vi "Interpolate R to T.vi"(7 "CHANNEL":i32, 8 "RESISTANCE (OHMS)":dbl, 9 "FILE INFO":T1(array[cluster]), 10 "R/T POINTS":cluster{dbl, dbl}[][](array[cluster]), 11 "CONFIGURATION CLUSTER":T2) -> (1 "TEMPERATURE":dbl, 2 "TEMPERATURE UNIT":string, 3 "UNMODIFIED CONFIGURATION CLUSTER":T2, 5 "R PAST CALIBRATION RANGE":bool)   [LabVIEW 2012]
doc: "Calculates temperature from the given\nor measured resistance. Uses the \nchannel's calibration curve for inter-\npolation."
panel:
  # "Interpolate R to T.vi"
  # "This is the \"direct temperature display VI\".  It requires the file info array of clusters and the R/T points 2-dimensional array of clusters. Both clusters are obtained by running \"read all RT calibration files.vi\". \n\nIndependent of the sign of the temperature coefficient of the sensor, the R values must be in ascending order. If the input value R is lower than R of the first breakpoint, or if it higher than the R of the last breakpoint, the first or last breakpoint temperature is returned and the \"R past calibration range\" indicator is set true.\n\nInstead of resistances, the calibration file can list breakpoints using log(R). This alternative must have been specified in the information file."
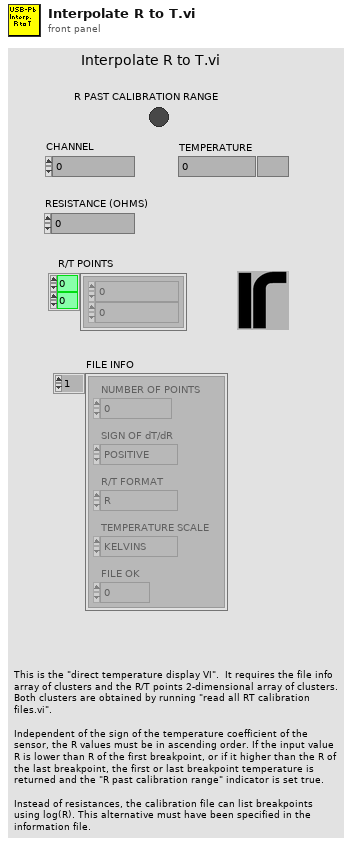
[diagram p1: front panel]
types:
  T1 = cluster{"NUMBER OF POINTS":i32, "SIGN OF dT/dR":enum16{"POSITIVE", "NEGATIVE"}, "R/T FORMAT ":enum16{"R", "LOG(R)"}, "TEMPERATURE SCALE":enum16{"KELVINS", "CELSIUS"}, "FILE OK":i32}[]
  T2 = cluster{"VISA RESOURCE":refnum<visa-resource-name>, "PICOBUS ADDRESS":u8, "DISABLE AL":u8, "REMOTE":u8, "INPUT":u8, "CHANNEL":u8, "RANGE":u8, "EXCITATION":u8, "DISPLAY":u8, "DIGITAL REFERENCE":u16, "SET POINT":dbl, "PROP GAIN":u8, "INTG":u8, "DERIV":u8, "POWER BIAS":u8, "POWER RANGE":u8, "INFO STRING":string, "HEATER RESISTANCE":dbl, "INTERVAL":u8, " SENSOR dR/dT":u8}
  T3 = cluster{"NUMBER OF POINTS":i32, "SIGN OF dT/dR":enum16{"POSITIVE", "NEGATIVE"}, "R/T FORMAT ":enum16{"R", "LOG(R)"}, "TEMPERATURE SCALE":enum16{"KELVINS", "CELSIUS"}, "FILE OK":i32}
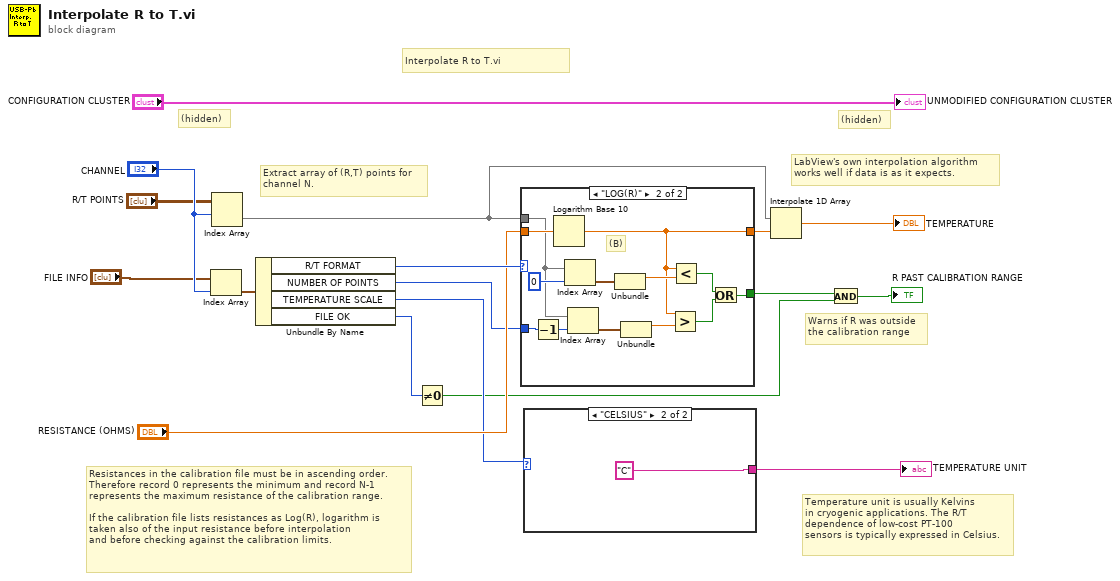
[diagram p0: block diagram]
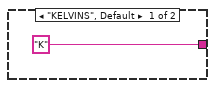
[diagram p2: hidden frame]
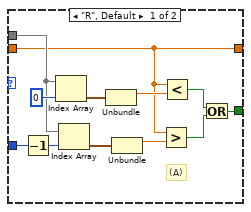
[diagram p3: hidden frame]
diagram:
  # "Resistances in the calibration file must be in ascending order.\nTherefore record 0 represents the minimum and record N-1\nrepresents the maximum resistance of the calibration range.\n\nIf the calibration file lists resistances as Log(R), logarithm is\ntaken also of the input resistance before interpolation\nand before checking against the calibration limits."
  # "LabView's own interpolation algorithm\nworks well if data is as it expects."
  # "Temperature unit is usually Kelvins\nin cryogenic applications. The R/T\ndependence of low-cost PT-100\nsensors is typically expressed in Celsius."
  # "Warns if R was outside\nthe calibration range"
  # "Extract array of (R,T) points for \nchannel N."
  # "(hidden)"
  # "(hidden)"
  # "Interpolate R to T.vi"
  n1 = Index Array(array="FILE INFO", index="CHANNEL") -> (element=w15:T3)
  n2 = Index Array(array="R/T POINTS", index (row)="CHANNEL") -> (element=w10:cluster{dbl, dbl}[])  [unwired: 1 in]
  n3 = Unbundle By Name(w15) -> ("R/T FORMAT"=w13:enum16{"R", "LOG(R)"}, "NUMBER OF POINTS"=w11:i32, "TEMPERATURE SCALE"=w8:enum16{"KELVINS", "CELSIUS"}, "FILE OK"=w5:i32)
  n4 = Not Equal To 0?(x=w5) -> (x != 0?=w1:bool)
  n5 = case shown="\"LOG(R)\"" w13 {
    tunnel: "RESISTANCE (OHMS)" -> [w19 w42]
    tunnel: [w19 w31] -> w14
    tunnel: w11 -> [w21 w33]
    tunnel: w10 -> [w20 w32]
    tunnel: [w18 w30] -> w3
    frame "R", Default {
      # "(A)"
      n6 = Decrement(x=w21) -> (x-1=w26:i32)
      n7 = Index Array(array=w20, index=0) -> (element=w27:cluster{dbl, dbl})
      n8 = Index Array(array=w20, index=w26) -> (element=w28:cluster{dbl, dbl})
      n9 = Unbundle(w27) -> (w23:dbl)  [unwired: 1 out]
      n10 = Unbundle(w28) -> (w22:dbl)  [unwired: 1 out]
      n11 = Greater?(x=w19, y=w22) -> (0:w24:bool)
      n12 = Less?(x=w19, y=w23) -> (x < y?=w25:bool)
      n13 = Or(x=w25, y=w24) -> (x .or. y?=w18:bool)
    }
    frame "LOG(R)" {
      # "(B)"
      n14 = Decrement(x=w33) -> (x-1=w37:i32)
      n15 = Logarithm Base 10(1:w42) -> (0:w31:dbl)
      n16 = Index Array(array=w32, index=0) -> (element=w36:cluster{dbl, dbl})
      n17 = Index Array(array=w32, index=w37) -> (element=w35:cluster{dbl, dbl})
      n18 = Unbundle(w36) -> (w40:dbl)  [unwired: 1 out]
      n19 = Unbundle(w35) -> (w41:dbl)  [unwired: 1 out]
      n20 = Greater?(x=w31, y=w41) -> (0:w39:bool)
      n21 = Less?(x=w31, y=w40) -> (x < y?=w38:bool)
      n22 = Or(x=w38, y=w39) -> (x .or. y?=w30:bool)
    }
  }
  n23 = case shown="\"CELSIUS\"" w8 {
    tunnel: ["K" "C"] -> w7
    frame "KELVINS", Default {
    }
    frame "CELSIUS" {
    }
  }
  "TEMPERATURE UNIT" <- w7
  n24 = Interpolate 1D Array(1:w14, 2:w10) -> (0:→"TEMPERATURE":dbl)
  n25 = And(x=w3, y=w1) -> (x .and. y?=→"R PAST CALIBRATION RANGE":bool)
  "UNMODIFIED CONFIGURATION CLUSTER" <- "CONFIGURATION CLUSTER"
